vi "Create Directory.vi"(8 "error in (no error)":errorcluster, 11 "Path In":path) -> (0 "error out":errorcluster, 3 "Directory":path)   [LabVIEW 2021, in "File_CIF_U.lvlib"]
doc: "Prune to the directory (if file path provided). Check if directory exists and create the directory if needed."
uses:
  File_CIF_U.lvlib
  <vilib>/Utility/error.llb/Clear Errors.vi
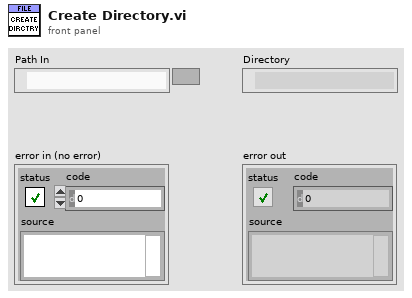
[diagram p1: front panel]
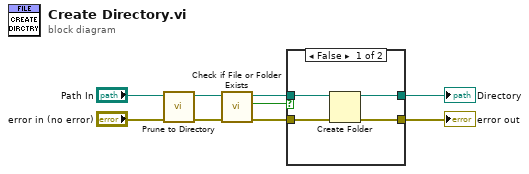
[diagram p0: block diagram]
diagram:
  n1 = call "Prune to Directory.vi"("error in (no error)"="error in (no error)", "Path In"="Path In") -> ("error out"=w3:errorcluster, "Directory"=w4:path)  [unwired: 8 in]
  n2 = call <vilib>:"Check if File or Folder Exists.vi"("error in (no error)"=w3, "path"=w4) -> ("error out"=w7:errorcluster, "file or folder exists?"=w9:bool, "dup path"=w8:path)  [unwired: 7 in]
  n3 = case shown="False" w9 {
    tunnel: w8 -> [w13 w15]
    tunnel: w7 -> [w12 w14]
    tunnel: [w11 w14] -> w5
    tunnel: [w10 w15] -> w6
    frame False {
      n4 = Create Folder(path (use dialog)=w13, error in=w12) -> (created path=w10:path, error out=w11:errorcluster)  [unwired: 1 in, 1 out]
    }
    frame True {
    }
  }
  "Directory" <- w6
  "error out" <- w5
